vi "L Vwrite read serial.vi"(5 "timoccur":i32, 6 "timeo":i32, 7 "bsize":i32, 9 "buf":i8[](array[numeric])=array[4097 elements], 10 "iswrite":i32, 11 "h":u32) -> (1 "buf out":i8[](array[numeric]), 2 "bytes w/r":i32, 3 "timoccur out":i32)   [LabVIEW 2010]
doc: "int LVwrite_read_serial(pserial_handle_t h, int iswrite,void*buf,int bsize,int timeo,int*timoccur);"
uses:
  <userlib>/libcommon_serial/libcommon_serial.so
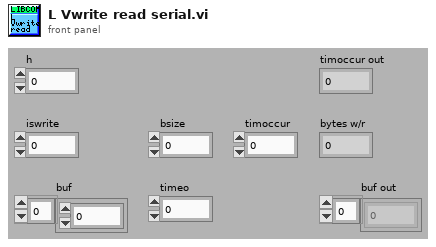
[diagram p1: front panel]
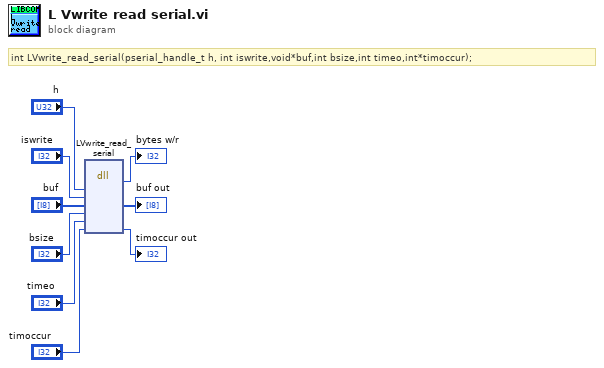
[diagram p0: block diagram]
diagram:
  # "int LVwrite_read_serial(pserial_handle_t h, int iswrite,void*buf,int bsize,int timeo,int*timoccur);"
  n1 = dll-call lib="usr/local/natinst/LabVIEW-2010/user.lib/libcommon_serial/libcommon_serial.*" fn="LVwrite_read_serial"("h"="h", "iswrite"="iswrite", "buf"="buf", "bsize"="bsize", "timeo"="timeo", "timoccur"="timoccur") -> ("return type"=→"bytes w/r":i32, "buf"=→"buf out":i8[], "timoccur"=→"timoccur out":i32)  [unwired: 7 in, 2 out]
